vi "kousei - Build POST Request Data.vi"(7 "Request ID":string, 8 "error in (no error)":errorcluster, 11 "Input Text":string) -> (0 "error out":errorcluster, 3 "JSON string":string)   [LabVIEW 2015, in "LV-Proof-Reading.lvlib"]
uses:
  LV-Proof-Reading.lvlib
  kousei - Post Data JSON.ctl
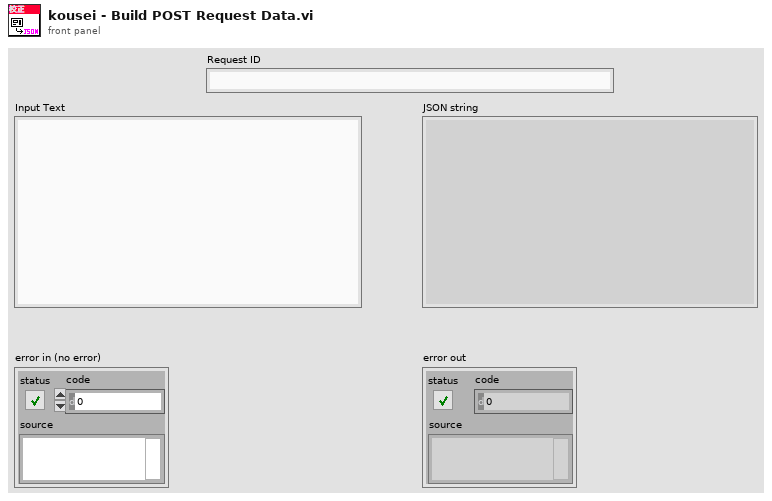
[diagram p1: front panel]
types:
  T1 = typedef "LV-Proof-Reading.lvlib/kousei - Post Data JSON.ctl" = cluster{"id":string, "jsonrpc":string, "method":string, "params":cluster{"q":string}}
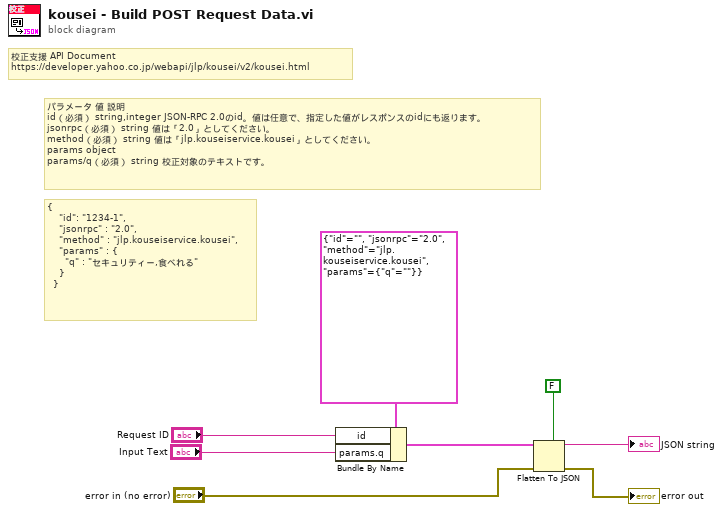
[diagram p0: block diagram]
diagram:
  # "校正支援 API Document\nhttps://developer.yahoo.co.jp/webapi/jlp/kousei/v2/kousei.html"
  # "{\n    \"id\": \"1234-1\",\n    \"jsonrpc\" : \"2.0\",\n    \"method\" : \"jlp.kouseiservice.kousei\",\n    \"params\" : {\n      \"q\" : \"セキュリティー,食べれる\"\n    }\n  }"
  # "パラメータ\t値\t説明\nid（必須）\tstring,integer\tJSON-RPC 2.0のid。値は任意で、指定した値がレスポンスのidにも返ります。\njsonrpc（必須）\tstring\t値は「2.0」としてください。\nmethod（必須）\tstring\t値は「jlp.kouseiservice.kousei」としてください。\nparams\tobject\t\nparams/q（必須）\tstring\t校正対象のテキストです。"
  n1 = Bundle By Name(cluster=T1 {"id"="", "jsonrpc"="2.0", "method"="jlp.kouseiservice.kousei", "params"={"q"=""}} ("JSON root object"), "id"="Request ID", "params.q"="Input Text") -> (w5:T1)
  n2 = Flatten To JSON(enable LabVIEW extensions? (T)=FALSE, anything=w5, error in (no error)="error in (no error)") -> (JSON string=→"JSON string":string, 11:→"error out":errorcluster)
